vi "出账写入数据库.vi"(10 "输出簇":T1) -> ()   [LabVIEW 2010]
panel:
  in  "error in (no error)":errorcluster caption="错误输入（无错误）"
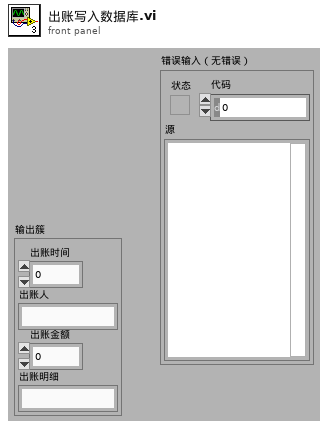
[diagram p1: front panel]
types:
  T1 = cluster{"出账时间":u64, "出账人":string, "出账金额":dbl, "出账明细":string}
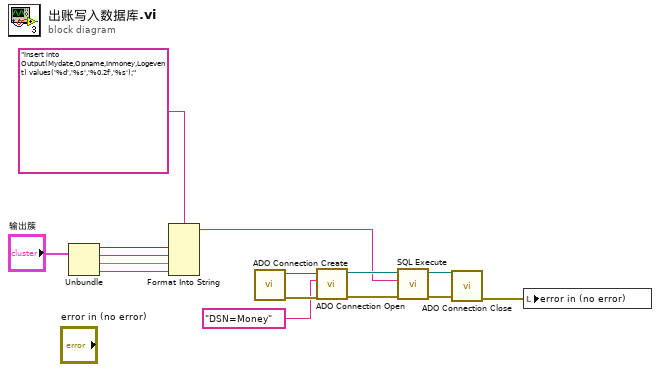
[diagram p0: block diagram]
diagram:
  n1 = Unbundle("输出簇") -> ("出账时间"=w1:u64, "出账人"=w6:string, "出账金额"=w5:dbl, "出账明细"=w4:string)
  n2 = Format Into String(format string="insert into Output(Mydate,Opname,Inmoney,Logevent) values('%d','%s','%0.2f','%s');", w1, w6, w5, w4) -> (resulting string=w2:string)  [unwired: 2 in, 1 out]
  n3 = call "ADO Connection Create.vi"() -> ("error out"=w15:errorcluster, "ADODB._Connection Out"=w14:refnum<k7>)  [unwired: 10 in]
  n4 = call "ADO Connection Open.vi"("error in (no error)"=w15, "ConnectionString"="DSN=Money", "ADODB._Connection In"=w14) -> ("error out"=w10:errorcluster, "ADODB._Connection Out"=w11:refnum<k7>)  [unwired: 7 in]
  n5 = call "SQL Execute.vi"("error in (no error)"=w10, "Command Text"=w2, "ADODB._Connection In"=w11) -> ("error out"=w8:errorcluster, "ADODB._Connection Out"=w9:refnum<k7>)  [unwired: 5 in, 2 out]
  n6 = call "ADO Connection Close.vi"("error in (no error)"=w8, "ADODB._Connection In"=w9) -> ("error out"=w12:errorcluster)  [unwired: 8 in, 1 out]
  n7 = local write "error in (no error)"(w12) -> ()
